vi "(SubVI) Title CB.vi"(1 "Talent CB":refnum<vi>, 2 "Basic info element":T1) -> ()   [LabVIEW 2024]
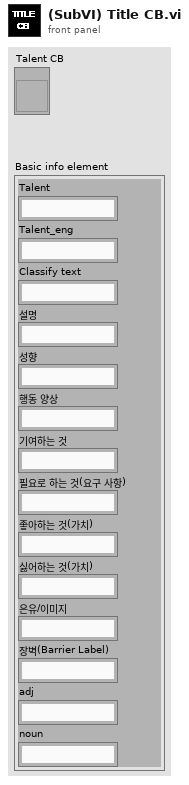
[diagram p1: front panel]
types:
  T1 = cluster{"Talent":string, "Talent_eng":string, "Classify text":string, "설명":string, "성향":string, "행동 양상":string, "기여하는 것":string, "필요로 하는 것(요구 사항)":string, "좋아하는 것(가치)":string, "싫어하는 것(가치)":string, "은유/이미지":string, "장벽(Barrier Label)":string, "adj":string, "noun":string}
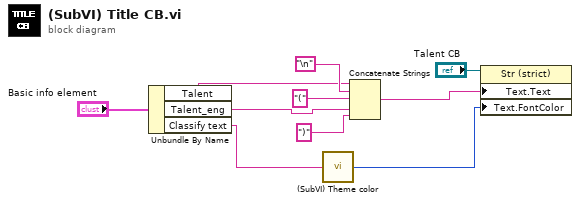
[diagram p0: block diagram]
diagram:
  n1 = Unbundle By Name("Basic info element") -> ("Talent"=w8:string, "Talent_eng"=w4:string, "Classify text"=w7:string)
  n2 = call "(SubVI) Theme color.vi"("Classify text"=w7) -> ("Classify color"=w1:u32)
  n3 = Concatenate Strings(w8, "\n", "(", w4, ")") -> (w5:string)
  n4 = property class="Str (strict)"(reference="Talent CB", "Text.Text"=w5, "Text.FontColor"=w1) -> ()  [unwired: 1 in, 2 out]
